vi "PDLM_GetFrequencyLimits.vi"(8 "error in (no error)":errorcluster, 11 "USBIdx":i32) -> (0 "error out":errorcluster, 1 "MaxFreq":u32, 2 "MinFreq":u32, 3 "return type":i32)   [LabVIEW 2019]
uses:
  <userlib>/TaikoLaser/PDLM_DllPath_global.vi
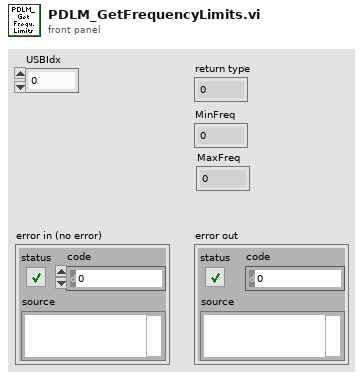
[diagram p1: front panel]
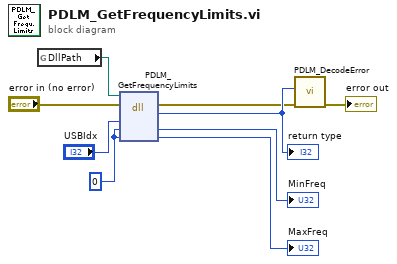
[diagram p0: block diagram]
diagram:
  w1 = u32 0 ("mode")
  n1 = global read "PDLM_DllPath_global.vi" "DllPath"() -> (w5:path)
  n2 = dll-call lib="M:/_dev/progs/LabVIEW/_lib/PQ/Taiko/pdlm_lib.dll" fn="PDLM_GetFrequencyLimits"(path in=w5, error in="error in (no error)", "USBIdx"="USBIdx", "MinFreq"=w1, "MaxFreq"=w1) -> (error out=w7:errorcluster, "return type"=w8:i32, "MinFreq"=→"MinFreq":u32, "MaxFreq"=→"MaxFreq":u32)  [unwired: 2 in, 1 out]
  "return type" <- w8
  n3 = call <userlib>:"PDLM_DecodeError.vi"("error in (no error)"=w7, "code"=w8) -> ("error out"=→"error out":errorcluster)  [unwired: 7 in, 2 out]
